vi "h5_write_waveform.vi"(7 "object name":string, 8 "error in":errorcluster, 9 "units (au)":string="au", 10 "waveform":waveform(dbl), 11 "h5 ref in":T1 format="%.0x") -> (0 "error out":errorcluster, 2 "duplicate waveform":waveform(dbl), 3 "dup h5 ref":T1 format="%.0x")   [LabVIEW 2015]
uses:
  <vilib>/addons/h5labview2/base/hid_t.ctl
  <vilib>/addons/h5labview2/attrib/H5A.lvlib
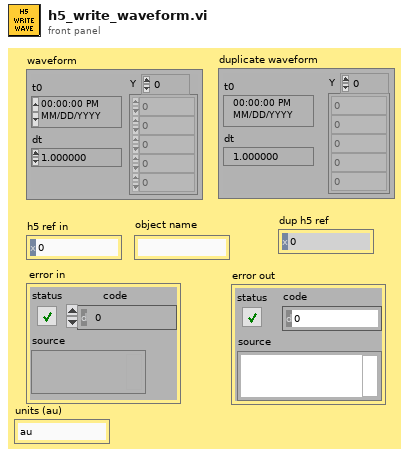
[diagram p1: front panel]
types:
  T1 = typedef "hid_t.ctl" = i32
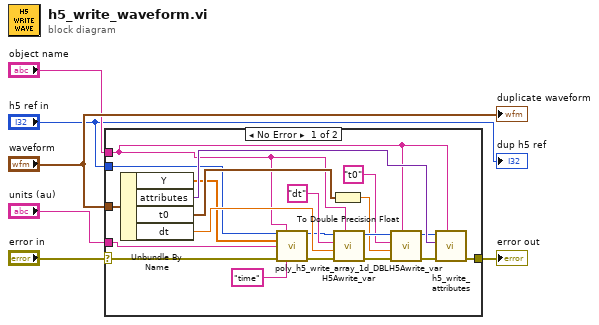
[diagram p0: block diagram]
diagram:
  n1 = case shown="No Error" "error in" {
    selector: "error in" -> [w10 w27]
    tunnel: "h5 ref in" -> [w12 _]
    tunnel: "waveform" -> [w26 _]
    tunnel: [w24 w27] -> w5
    tunnel: "object name" -> [w13 _]
    tunnel: "units (au)" -> [w7 _]
    frame No Error {
      n2 = Unbundle By Name(w26) -> ("Y"=w14:dbl[], "attributes"=w25:variant, "t0"=w17:timestamp, "dt"=w15:dbl)
      n3 = call "poly_h5_write_array_1d_DBL.vi"("h5 dir ref"=w12, "dataset name"=w13, "array"=w14, "units (au)"=w7, "error in (no error)"=w10, "dim (index)"="time") -> ("h5 obj ref"=w11:i32, "error out"=w9:errorcluster)  [unwired: 8 in]
      n4 = To Double Precision Float(number=w17) -> (double precision float=w16:dbl)
      n5 = call <vilib>:"H5Awrite_var.vi"("object name"=w13, "error in (no error)"=w9, "data"=w15, "attrib name"="dt", "ref in"=w11) -> ("error out"=w21:errorcluster, "ref out"=w22:T1)  [unwired: 4 in, 1 out]
      n6 = call <vilib>:"H5Awrite_var.vi"("object name"=w13, "error in (no error)"=w21, "data"=w16, "attrib name"="t0", "ref in"=w22) -> ("error out"=w20:errorcluster, "ref out"=w19:T1)  [unwired: 4 in, 1 out]
      n7 = call "h5_write_attributes.vi"("object name"=w13, "error in"=w20, "attributes"=w25, "h5 ref"=w19) -> ("error out"=w24:errorcluster)  [unwired: 6 in, 1 out]
    }
    frame Error {
    }
  }
  "error out" <- w5
  "duplicate waveform" <- "waveform"
  "dup h5 ref" <- "h5 ref in"
